vi "Main.vi"   [LabVIEW 2020, in "Display As.lvlib"]
uses:
  Display As.lvlib
  DA Child A/DA Child A.lvclass
  C:/dev/lv/2020/lv-oopanel/Examples/Display As/DA Parent/DA Parent.lvclass
  DA Child B/DA Child B.lvclass
  DA Parent/DA Parent.lvclass
  C:/dev/lv/2020/lv-oopanel/OOPanel/ArrayPanel/ArrayPanel.lvclass
  OOPanel/ArrayManager/ArrayManager.lvclass
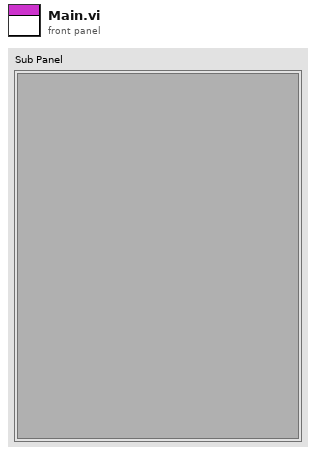
[diagram p1: front panel]
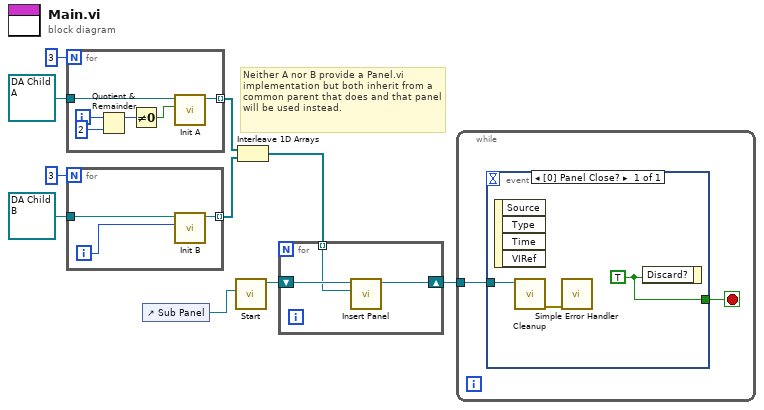
[diagram p0: block diagram]
diagram:
  # "Neither A nor B provide a Panel.vi implementation but both inherit from a common parent that does and that panel will be used instead."
  n1 = for {
    N: 3 -> [_]
    tunnel: refnum<class "DA Child A.lvclass"> refnum ("Display As.lvlib:DA Child A.lvclass") -> [w13]
    tunnel: [w11] -> w4 mode=indexing
    i -> [w16]
    n2 = Quotient & Remainder(x=w16, y=2) -> (x-y*floor(x/y)=w14:i32)  [unwired: 1 out]
    n3 = Not Equal To 0?(x=w14) -> (x != 0?=w12:bool)
    n4 = call "Init A.vi"("Boolean"=w12, "DA Child A in"=w13) -> ("DA Child A out"=w11:refnum<class "DA Child A.lvclass">)  [unwired: 8 in, 1 out]
  }
  n5 = for {
    N: 3 -> [_]
    tunnel: refnum<class "DA Child B.lvclass"> refnum ("Display As.lvlib:DA Child B.lvclass") -> [w19]
    tunnel: [w17] -> w3 mode=indexing
    i -> [w18]
    n6 = call "Init B.vi"("Numeric"=w18, "DA Child B in"=w19) -> ("DA Child B out"=w17:refnum<class "DA Child B.lvclass">)  [unwired: 8 in, 1 out]
  }
  n7 = control-ref of="Sub Panel"() -> (w10:refnum<vi>)
  n8 = call "Start.vi"("Container"=w10) -> ("ArrayManager out"=w9:refnum<class "ArrayManager.lvclass">)  [unwired: 9 in, 1 out]
  n9 = Interleave 1D Arrays(w4, w3) -> (w2:refnum<class "DA Parent.lvclass">[])
  n10 = for {
    shift-right: [w20] -> w1
    shift-left: w9 -> [w22]
    tunnel: w2 -> [w21] mode=indexing
    n11 = call "Insert Panel.vi"("Panel/Type"=w21, "PanelArray in"=w22) -> ("PanelArray out"=w20:refnum<class "ArrayManager.lvclass">)  [unwired: 7 in, 2 out]
  }
  n12 = while {
    tunnel: w1 -> [w24]
    stop <- w23 stop-if-true
    n13 = event shown="[0] Panel Close?" {
      selector: _ -> [_]
      dyn-events: _ -> [_]
      timeout: _ -> [_]
      tunnel: w24 -> [w26]
      tunnel: [w27] -> w23
      event Panel Close? {
        w27 = TRUE
        n14 = event-data() -> ()  [unwired: 1 in, 4 out]
        n15 = call "Cleanup.vi"("PanelArray in"=w26) -> ("error out"=w25:errorcluster)  [unwired: 10 in]
        n16 = call <vilib>:"Simple Error Handler.vi"("error in (no error)"=w25) -> ()  [unwired: 4 in, 5 out]
        n17 = event-data("Discard?"=w27) -> ()  [unwired: 1 in, 1 out]
      }
    }
  }
